vi "Link Async Parameters.vi"(7 "Parameter R Table":refnum<class "Registry.lvclass">, 8 "error in (no error)":errorcluster, 9 "Async Payload":T1 {"Trigger Command" format="%04x"; "Data" format="%04x"; "Data Address" format="%04x"; "Configuration" format="%04x"; "Configuration Address" format="%04x"}, 10 "Parameter W Table":refnum<class "Registry.lvclass">, 11 "Async RT-RT Message in":refnum<class "Async RT-RT Message.lvclass">) -> (0 "error out":errorcluster, 2 "Parameter W Table out":refnum<class "Registry.lvclass">, 3 "Async RT-RT Message out":refnum<class "Async RT-RT Message.lvclass">, 5 "Parameter R Table out":refnum<class "Registry.lvclass">)   [LabVIEW 2020, in "BCI-1553 API.lvlib" / "Async RT-RT Message.lvclass"]
doc: "<DO NOT CALL>\n\nOverrides the default asynchronous Message parameter linking. An RT-RT message doesn't transact any data to or from the Bus Controller, so it cannot have any specific parameters."
uses:
  Async RT-RT Message.lvclass
  Dependencies/Registry/Registry.lvclass
  TypeDefs/Async Payload.ctl
  BCI-1553 API.lvlib
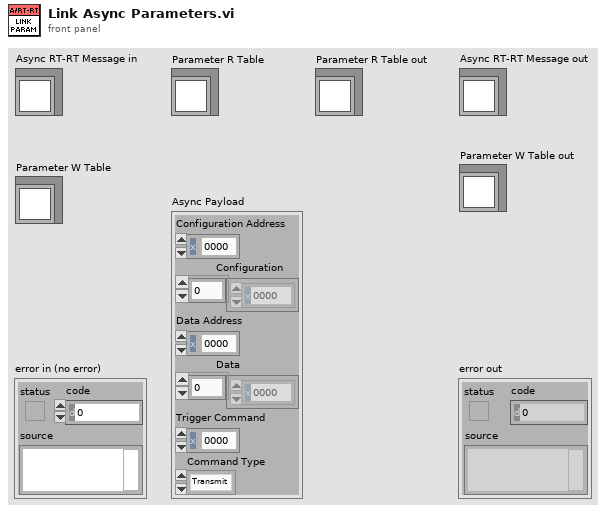
[diagram p1: front panel]
types:
  T1 = typedef "BCI-1553 API.lvlib/Async Payload.ctl" = cluster{"Configuration Address":u16, "Configuration":u16[], "Data Address":u16, "Data":u16[], "Trigger Command":u16, "Command Type":enum16{"Transmit", "Receive"}}
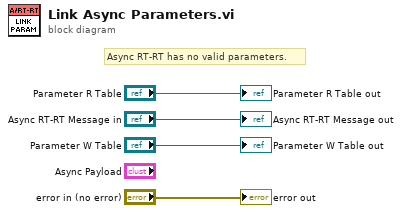
[diagram p0: block diagram]
diagram:
  # "Async RT-RT has no valid parameters."
  "error out" <- "error in (no error)"
  "Async RT-RT Message out" <- "Async RT-RT Message in"
  "Parameter R Table out" <- "Parameter R Table"
  "Parameter W Table out" <- "Parameter W Table"
